vi "Write to Refnum Table.vi"(8 "ControlIndex":i32, 9 "ClassName":string, 10 "Control Refnum":refnum<vi>, 11 "Typed Refnum Table In":variant) -> (3 "Typed Refnum Table Out":variant)   [LabVIEW 2015, in "ActorEvents.lvlib" / "ActorAutoRegistration.lvclass"]
uses:
  ActorAutoRegistration.lvclass
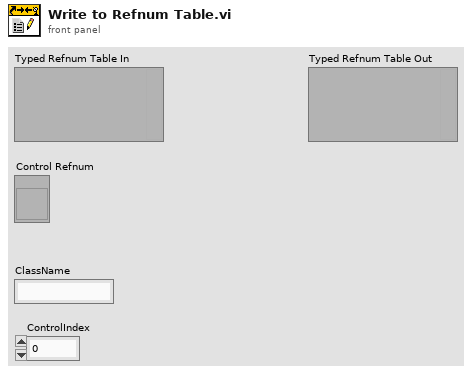
[diagram p1: front panel]
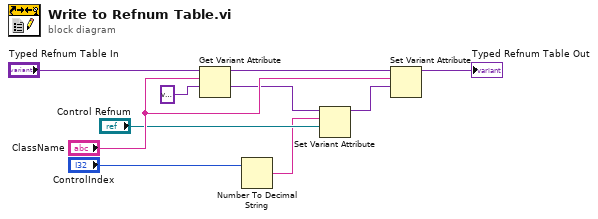
[diagram p0: block diagram]
diagram:
  n1 = Get Variant Attribute(Variant="Typed Refnum Table In", name="ClassName", default value (empty Variant)=variant ("default value (empty variant)")) -> (duplicate Variant=w7:variant, value=w3:variant)  [unwired: 1 in, 2 out]
  n2 = Number To Decimal String(number="ControlIndex") -> (decimal integer string=w5:string)  [unwired: 1 in]
  n3 = Set Variant Attribute(Variant=w3, name=w5, value="Control Refnum") -> (Variant out=w8:variant)  [unwired: 1 in, 2 out]
  n4 = Set Variant Attribute(Variant=w7, name="ClassName", value=w8) -> (Variant out=→"Typed Refnum Table Out":variant)  [unwired: 1 in, 2 out]
